vi "Write sub-VI.vi"(7 "Port to Write (RT)":enum8{"1", "2", "3", "4"}(ring) caption="Port", 8 "Write sub-VI Error In":errorcluster, 9 "Write Data?":bool, 10 "String To Write":string, 11 "FPGA VI Reference":refnum<k20>) -> (0 "Write sub-VI Error Out":errorcluster, 1 "bytes to send":dbl, 3 "FPGA VI Reference Out":refnum<k20>)   [LabVIEW 2011]
doc: "Writes the data from the \"String To Write\" String Control to the WRITE_FIFO hosted on the FPGA when the \"Write Data\" button is pressed."
uses:
  <vilib>/rvi/errors/niLvFpgaMergeErrorWithErrorCode.vi
  <vilib>/rvi/errors/niLvFpgaAdjustHostInterfaceError.vi
  <vilib>/rvi/interface/nirviReadWriteControl/nirviReadWriteControl.xnode
  FPGA Bitfiles/AURLabROVControl_FPGATarget_9870InterfaceDMA_6DB679DB.lvbitx
  cRIO/FPGA/9870 Interface DMA (FPGA).vi
  <vilib>/rvi/interface/nirviMethod/nirviMethod.xnode
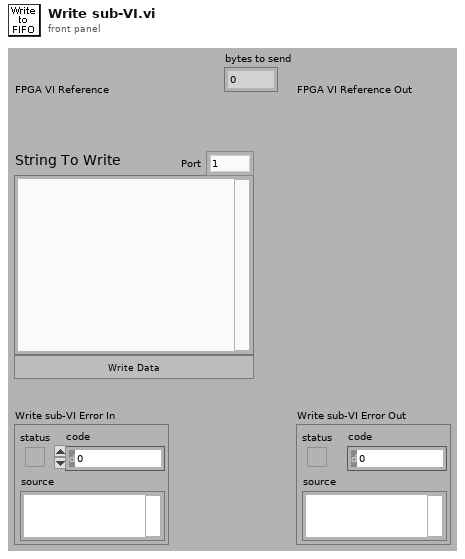
[diagram p1: front panel]
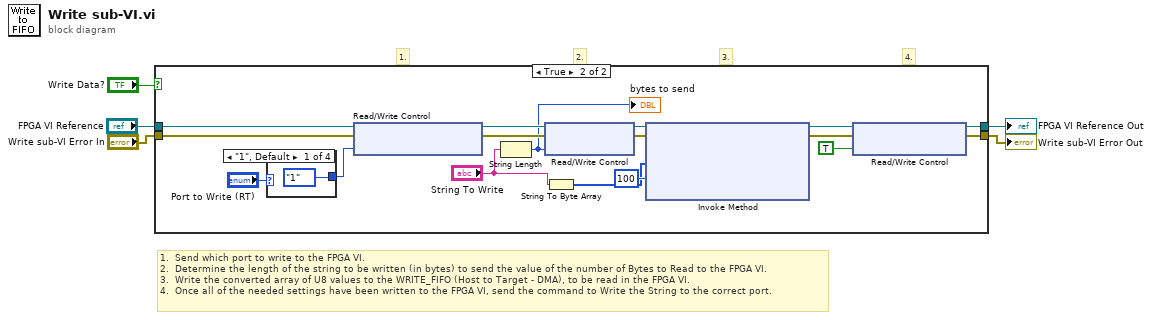
[diagram p0: block diagram]
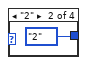
[diagram p3: hidden frame]
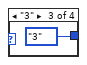
[diagram p4: hidden frame]
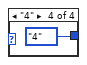
[diagram p5: hidden frame]
diagram:
  # "1.  Send which port to write to the FPGA VI.\n2.  Determine the length of the string to be written (in bytes) to send the value of the number of Bytes to Read to the FPGA VI.\n3.  Write the converted array of U8 values to the WRITE_FIFO (Host to Target - DMA), to be read in the FPGA VI.\n4.  Once all of the needed settings have been written to the FPGA VI, send the command to Write the String to the correct port."
  # "4."
  # "3."
  # "2."
  # "1."
  n1 = case shown="True" "Write Data?" {
    tunnel: "FPGA VI Reference" -> [w7 w17]
    tunnel: [w7 w20] -> w1
    tunnel: "Write sub-VI Error In" -> [w6 w16]
    tunnel: [w6 w21] -> w3
    frame False {
    }
    frame True {
      n2 = case shown="\"1\", Default" "Port to Write (RT)" {
        tunnel: [enum8{"0", "1", "2", "3", "4"}."1" ("Port To Write (FPGA)") enum8{"0", "1", "2", "3", "4"}."2" ("Port To Write (FPGA)") enum8{"0", "1", "2", "3", "4"}."3" ("Port To Write (FPGA)") enum8{"0", "1", "2", "3", "4"}."4" ("Port To Write (FPGA)")] -> w11
        frame "1", Default {
        }
        frame "2" {
        }
        frame "3" {
        }
        frame "4" {
        }
      }
      n3 = xnode "Read/Write Control"("FPGA VI Reference In"=w17, "error in"=w16, "Port To Write (FPGA)"=w11) -> ("FPGA VI Reference Out"=w18:refnum<k20>, "error out"=w19:errorcluster)
      n4 = String Length(string="String To Write") -> (length=w10:i32)
      "bytes to send" <- w10
      n5 = xnode "Read/Write Control"("FPGA VI Reference In"=w18, "error in"=w19, "Bytes to Send"=w10) -> ("FPGA VI Reference Out"=w14:refnum<k20>, "error out"=w15:errorcluster)
      n6 = String To Byte Array(string="String To Write") -> (unsigned byte array=w9:u8[])
      n7 = xnode "Invoke Method"("FPGA VI Reference In"=w14, "error in"=w15, "Data"=w9, "Timeout (ms)"=100) -> ("FPGA VI Reference Out"=w23:refnum<k20>, "error out"=w22:errorcluster)  [unwired: 1 out]
      n8 = xnode "Read/Write Control"("FPGA VI Reference In"=w23, "error in"=w22, "Write Data (FPGA)"=TRUE) -> ("FPGA VI Reference Out"=w20:refnum<k20>, "error out"=w21:errorcluster)
    }
  }
  "Write sub-VI Error Out" <- w3
  "FPGA VI Reference Out" <- w1
